vi "FSM Break In.vi"(4 "Abort":refnum<vi>, 6 "Dialog Indicator":refnum<vi>, 8 "error in (no error)":errorcluster, 9 "Break in Thr [MOhm]":refnum<vi>, 10 "Pressure Controls":T1, 11 "Signals":T2) -> (0 "error out":errorcluster, 2 "Aborted":bool)   [LabVIEW 2012, in "Autopatcher Daemon.lvlib"]
uses:
  Autopatcher Daemon.lvlib
panel:
  in  "Dialog Indicator 3":refnum<vi>
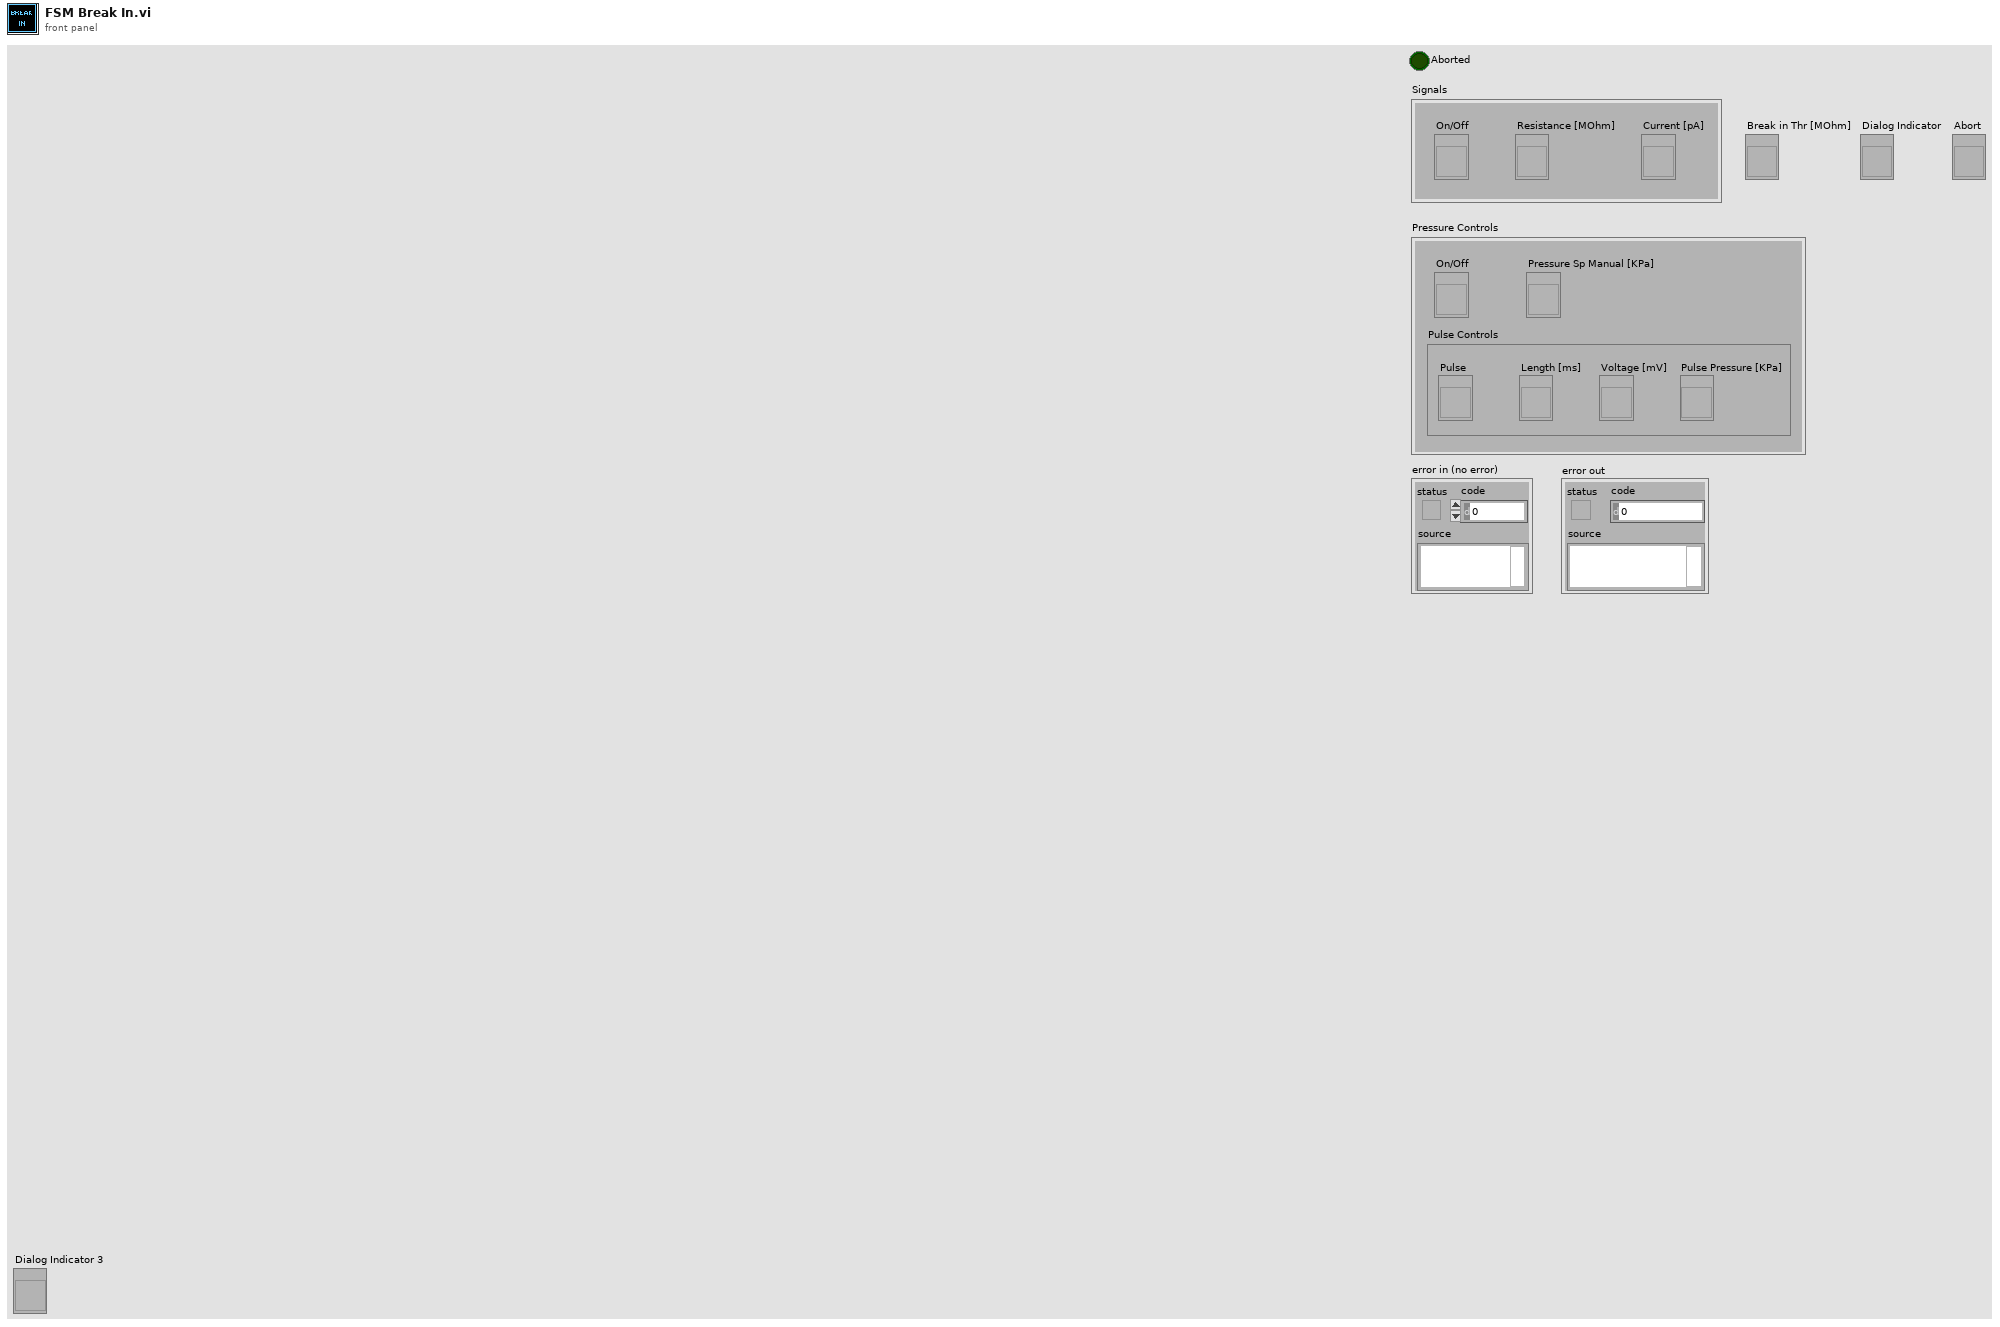
[diagram p1: front panel]
types:
  T1 = cluster{"On/Off":refnum<vi>, "Pulse Controls":cluster{"Pulse":refnum<vi>, "Length [ms]":refnum<vi>, "Voltage [mV]":refnum<vi>, "Pulse Pressure [KPa]":refnum<vi>}, "Pressure Sp Manual [KPa]":refnum<vi>}
  T2 = cluster{"On/Off":refnum<vi>, "Resistance [MOhm]":refnum<vi>, "Current [pA]":refnum<vi>}
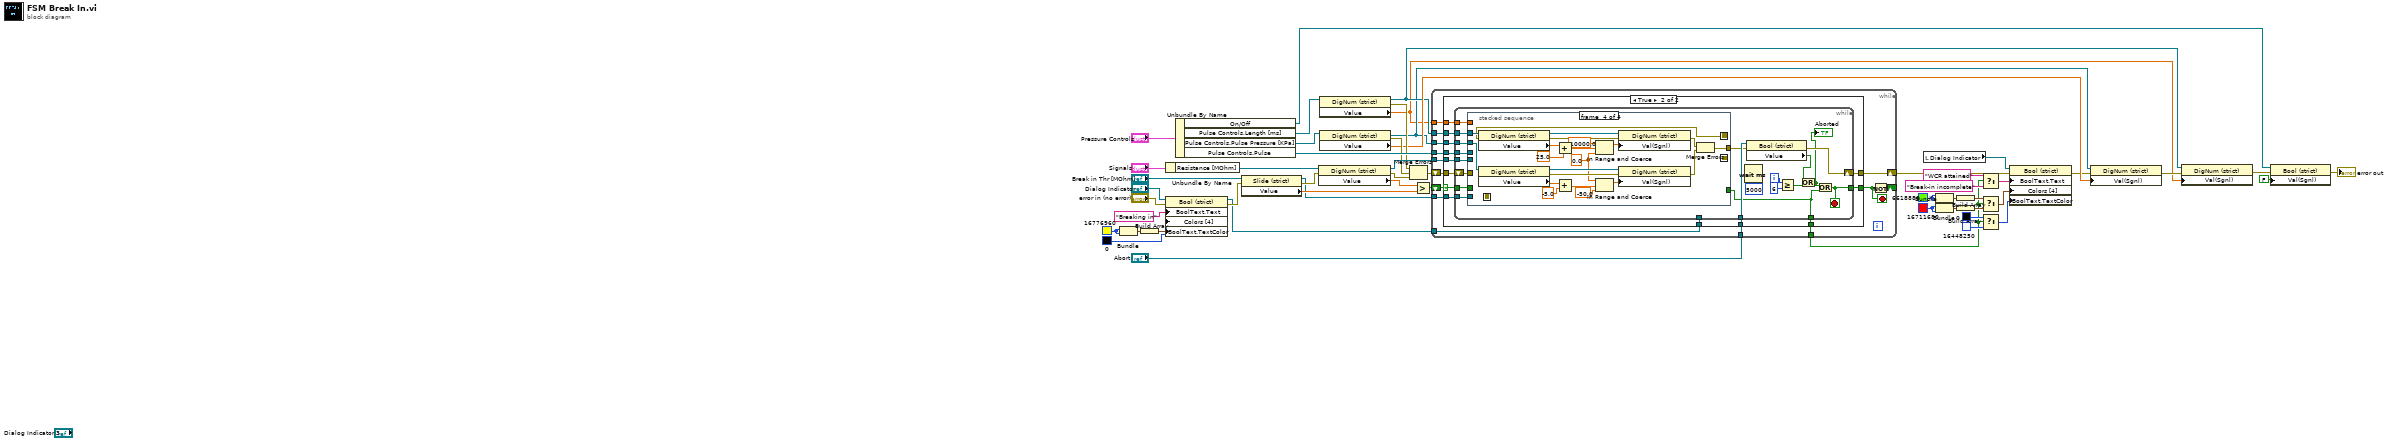
[diagram p0: block diagram]
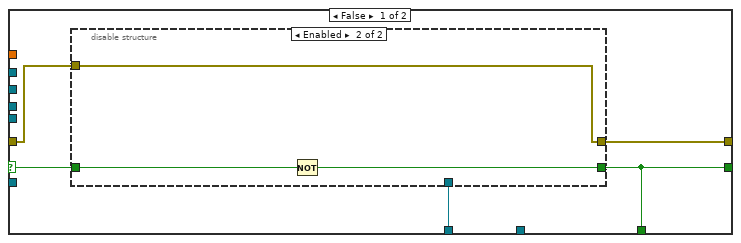
[diagram p2: hidden frame]
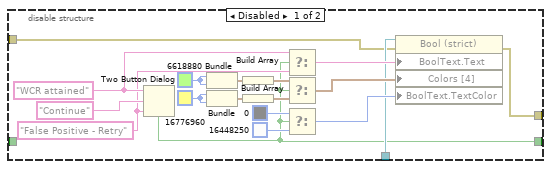
[diagram p3: hidden frame]
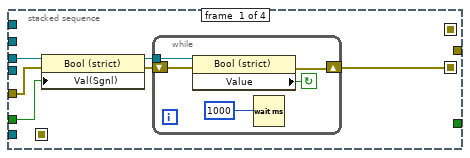
[diagram p4: hidden frame]
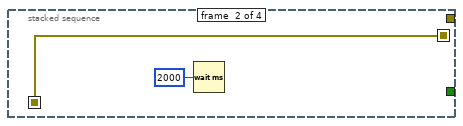
[diagram p5: hidden frame]
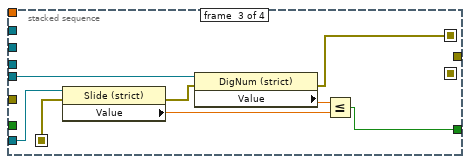
[diagram p6: hidden frame]
diagram:
  w16 = u32 6618880
  w14 = u32 16711680
  w41 = u32 16776960
  n1 = Bundle(w41, w41) -> (w38:cluster{u32, u32})  [unwired: 1 in]
  n2 = Build Array(w38) -> (w39:cluster{u32, u32}[])
  n3 = Unbundle By Name("Signals") -> ("Resistance [MOhm]"=w51:refnum<vi>)
  n4 = property class="Bool (strict)"(reference="Dialog Indicator", error in="error in (no error)", "BoolText.Text"="Breaking in" ("Boolean Text.Text"), "Colors [4]"=w39, "BoolText.TextColor"=u32 0) -> (reference out=w33:refnum<vi>, error out=w36:errorcluster)
  n5 = Unbundle By Name("Pressure Controls") -> ("On/Off"=w32:refnum<vi>, "Pulse Controls.Length [ms]"=w29:refnum<vi>, "Pulse Controls.Pulse Pressure [KPa]"=w30:refnum<vi>, "Pulse Controls.Pulse"=w46:refnum<vi>)
  n6 = property class="Slide (strict)"(reference="Break in Thr [MOhm]", error in=w36) -> (reference out=w47:refnum<vi>, error out=w49:errorcluster, "Value"=w53:dbl)
  n7 = property class="DigNum (strict)"(reference=w51, error in=w49) -> (reference out=w48:refnum<vi>, error out=w27:errorcluster, "Value"=w52:dbl)
  n8 = property class="DigNum (strict)"(reference=w29) -> (reference out=w23:refnum<vi>, error out=w25:errorcluster, "Value"=w1:dbl)  [unwired: 1 in]
  n9 = property class="DigNum (strict)"(reference=w30) -> (reference out=w21:refnum<vi>, error out=w26:errorcluster, "Value"=w24:dbl)  [unwired: 1 in]
  n10 = Merge Errors(w25, w26, w27) -> (w28:errorcluster)
  n11 = Greater?(x=w52, y=w53) -> (0:w50:bool)
  n12 = while {
    tunnel: w48 -> [w66]
    tunnel: w47 -> [w64]
    tunnel: w46 -> [w63]
    shift-right: [w60] -> _
    shift-left: w50 -> [w67]
    shift-right: [w62] -> w4
    shift-left: w28 -> [w65]
    tunnel: w33 -> [w59]
    tunnel: w21 -> [w58]
    tunnel: w23 -> [w57]
    tunnel: "Abort" -> [w56]
    tunnel: [w55] -> w5
    tunnel: w1 -> [w54]
    stop <- w61 stop-if-true
    n13 = case shown="True" w67 {
      selector: w67 -> [w69 w103]
      tunnel: w66 -> [_ w105]
      tunnel: w65 -> [w71 w106]
      tunnel: w64 -> [_ w104]
      tunnel: w63 -> [_ w102]
      tunnel: [w68 w101] -> w61
      tunnel: [w70 w100] -> w62
      tunnel: w59 -> [w72 w99]
      tunnel: w58 -> [_ w98]
      tunnel: w57 -> [_ w97]
      tunnel: w56 -> [_ w96]
      tunnel: [w68 w95] -> w55
      tunnel: w54 -> [_ w94]
      frame False {
        n14 = disable-structure shown="Enabled" {
          disable-tunnel: w72 -> [w76 _]
          disable-tunnel: w71 -> [w75 w91]
          disable-tunnel: [w74 w91] -> w70
          disable-tunnel: [w73 w92] -> w68
          disable-tunnel: w69 -> [_ w93]
          frame Disabled {
            w83 = u32 6618880
            w85 = u32 16776960
            w88 = "False Positive - Retry" ("Center Button Text (\"No\")")
            w89 = "WCR attained" ("message")
            n15 = Two Button Dialog(message=w89, 1:w88, 2:"Continue" ("T button name (\"OK\")")) -> (T button?=w73:bool)
            n16 = Bundle(w83, w83) -> (w82:cluster{u32, u32})  [unwired: 1 in]
            n17 = Bundle(w85, w85) -> (w84:cluster{u32, u32})  [unwired: 1 in]
            n18 = Build Array(w82) -> (w81:cluster{u32, u32}[])
            n19 = Build Array(w84) -> (w80:cluster{u32, u32}[])
            n20 = Select(t=w89, s=w73, f=w88) -> (s? t:f=w79:string)
            n21 = Select(t=w81, s=w73, f=w80) -> (s? t:f=w78:cluster{u32, u32}[])
            n22 = Select(t=u32 0, s=w73, f=u32 16448250) -> (s? t:f=w77:u32)
            n23 = property class="Bool (strict)"(reference=w76, error in=w75, "BoolText.Text"=w79, "Colors [4]"=w78, "BoolText.TextColor"=w77) -> (error out=w74:errorcluster)  [unwired: 1 out]
          }
          frame Enabled {
            n24 = Not(x=w93) -> (.not. x?=w92:bool)
          }
        }
      }
      frame True {
        n25 = while {
          tunnel: w105 -> [w124]
          tunnel: w104 -> [w123]
          tunnel: w103 -> [w122]
          tunnel: w102 -> [w121]
          tunnel: w96 -> [w120]
          shift-right: [w118] -> w100
          shift-left: w106 -> [w125]
          tunnel: [w119] -> w101
          tunnel: w99 -> [_]
          tunnel: w98 -> [w117]
          tunnel: w97 -> [w116]
          tunnel: [w114] -> w95
          tunnel: w94 -> [w112]
          i -> [w111]
          stop <- w119 stop-if-true
          n26 = stacked-sequence {
            seq-local: [w128 _ _ _] -> [_ w137 _ _]
            seq-local: [_ w137 _ _] -> [_ _ w141 _]
            seq-local: [_ _ w139 _] -> [_ _ _ w155]
            tunnel: w123 -> [_ _ w142 _]
            tunnel: w125 -> [w126 _ _ _]
            tunnel: w124 -> [_ _ w143 _]
            tunnel: w122 -> [w129 _ _ _]
            tunnel: w121 -> [w127 _ _ _]
            tunnel: [_ _ w140 _] -> w114
            tunnel: w117 -> [_ _ _ w166]
            tunnel: w116 -> [_ _ _ w167]
            tunnel: [_ _ _ w156] -> w115
            tunnel: w112 -> [_ _ _ _]
            frame #0 {
              n27 = property class="Bool (strict)"(reference=w127, error in=w126, "Val(Sgnl)"=w129) -> (reference out=w131:refnum<vi>, error out=w130:errorcluster)
              n28 = while {
                tunnel: w131 -> [w135]
                shift-right: [w132] -> w128
                shift-left: w130 -> [w134]
                stop <- w136 continue-if-true
                n29 = property class="Bool (strict)"(reference=w135, error in=w134) -> (error out=w132:errorcluster, "Value"=w136:bool)  [unwired: 1 out]
                n30 = Wait (ms)(milliseconds to wait=u32 1000 ("millisecond multiple")) -> ()  [unwired: 1 out]
              }
            }
            frame #1 {
              n31 = Wait (ms)(milliseconds to wait=u32 2000) -> ()  [unwired: 1 out]
            }
            frame #2 {
              n32 = property class="Slide (strict)"(reference=w142, error in=w141) -> (error out=w144:errorcluster, "Value"=w145:dbl)  [unwired: 1 out]
              n33 = property class="DigNum (strict)"(reference=w143, error in=w144) -> (error out=w139:errorcluster, "Value"=w146:dbl)  [unwired: 1 out]
              n34 = Less Or Equal?(x=w146, y=w145) -> (x <= y?=w140:bool)
            }
            frame #3 {
              w151 = 0.0 ("lower limit")
              n35 = property class="DigNum (strict)"(reference=w167, error in=w155) -> (reference out=w165:refnum<vi>, error out=w164:errorcluster, "Value"=w159:dbl)
              n36 = property class="DigNum (strict)"(reference=w166) -> (reference out=w163:refnum<vi>, error out=w162:errorcluster, "Value"=w158:dbl)  [unwired: 1 in]
              n37 = Add(x=w159, y=25.0) -> (x+y=w147:dbl)
              n38 = Add(x=w158, y=-5.0) -> (x+y=w154:dbl)
              n39 = In Range and Coerce(upper limit=10000.0, x=w147, lower limit=w151) -> (coerced(x)=w152:dbl)  [unwired: 1 out]
              n40 = In Range and Coerce(upper limit=w151, x=w154, lower limit=-50.0) -> (coerced(x)=w153:dbl)  [unwired: 1 out]
              n41 = property class="DigNum (strict)"(reference=w165, error in=w164, "Val(Sgnl)"=w152) -> (error out=w161:errorcluster)  [unwired: 1 out]
              n42 = property class="DigNum (strict)"(reference=w163, error in=w162, "Val(Sgnl)"=w153) -> (error out=w160:errorcluster)  [unwired: 1 out]
              n43 = Merge Errors(w161, w160) -> (w156:errorcluster)
            }
          }
          n44 = Wait (ms)(milliseconds to wait=u32 5000 ("millisecond multiple")) -> ()  [unwired: 1 out]
          n45 = property class="Bool (strict)"(reference=w120, error in=w115) -> (error out=w118:errorcluster, "Value"=w109:bool)  [unwired: 1 out]
          n46 = Greater Or Equal?(x=w111, y=6) -> (x >= y?=w108:bool)
          n47 = Or(x=w109, y=w108) -> (x .or. y?=w107:bool)
          "Aborted" <- w107
          n48 = Or(x=w107, y=w114) -> (x .or. y?=w119:bool)
        }
      }
    }
    n49 = Not(x=w61) -> (.not. x?=w60:bool)
  }
  n50 = local read "Dialog Indicator"() -> (w2:refnum<vi>)
  n51 = Bundle(w16, w16) -> (w17:cluster{u32, u32})  [unwired: 1 in]
  n52 = Bundle(w14, w14) -> (w15:cluster{u32, u32})  [unwired: 1 in]
  n53 = Build Array(w17) -> (w18:cluster{u32, u32}[])
  n54 = Build Array(w15) -> (w19:cluster{u32, u32}[])
  n55 = Select(t="WCR attained" ("message"), s=w5, f="Break-in incomplete" ("Center Button Text (\"No\")")) -> (s? t:f=w9:string)
  n56 = Select(t=w18, s=w5, f=w19) -> (s? t:f=w6:cluster{u32, u32}[])
  n57 = Select(t=u32 0, s=w5, f=u32 16448250) -> (s? t:f=w8:u32)
  n58 = property class="Bool (strict)"(reference=w2, error in=w4, "BoolText.Text"=w9, "Colors [4]"=w6, "BoolText.TextColor"=w8) -> (error out=w3:errorcluster)  [unwired: 1 out]
  n59 = property class="DigNum (strict)"(reference=w21, error in=w3, "Val(Sgnl)"=w24) -> (error out=w22:errorcluster)  [unwired: 1 out]
  n60 = property class="DigNum (strict)"(reference=w23, error in=w22, "Val(Sgnl)"=w1) -> (error out=w20:errorcluster)  [unwired: 1 out]
  n61 = property class="Bool (strict)"(reference=w32, error in=w20, "Val(Sgnl)"=FALSE ("Value")) -> (error out=→"error out":errorcluster)  [unwired: 1 out]
